vi "PCO_GetDeviceStatus.vi"(8 "error in (no error)":errorcluster {"code" format="%x"}, 10 "wNum":u16, 11 "ph":u64) -> (0 "error out":errorcluster {"code" format="%x"}, 1 "dwStatus":u32[](array[numeric]) format="%x", 2 "ErrorMessage":i32 format="%x", 3 "ph out":u64)   [LabVIEW 2019, in "SDK.lvlib" / "CameraAccess.lvlib"]
doc: "Gets the device availability status. Also returns the generation count if an IEEE 1394 interface is connected.\n\n dwStatus[0]-> 0x80000000: Device is available (0: not available)\ndwStatus[1]-> Generation count for IEEE1394 (undefined for other interfaces)"
uses:
  CameraAccess.lvlib
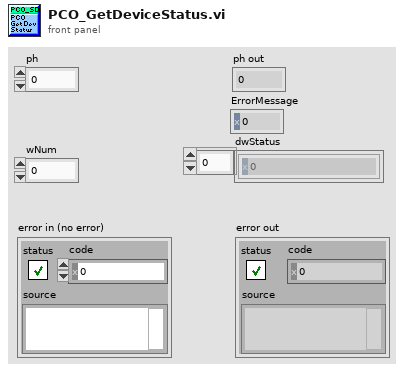
[diagram p1: front panel]
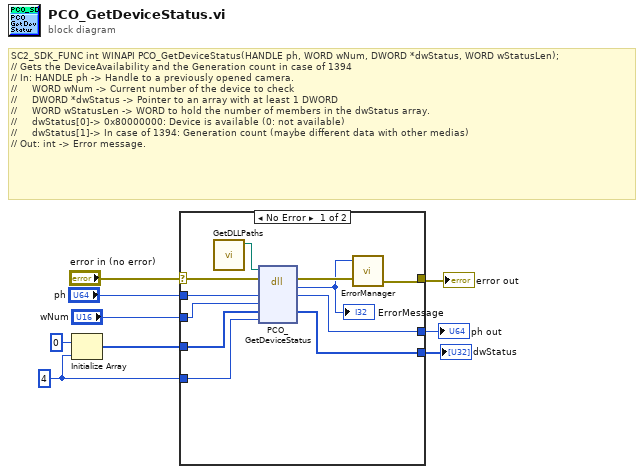
[diagram p0: block diagram]
diagram:
  w3 = u16 4 ("dimension size")
  # "SC2_SDK_FUNC int WINAPI PCO_GetDeviceStatus(HANDLE ph, WORD wNum, DWORD *dwStatus, WORD wStatusLen);\n// Gets the DeviceAvailability and the Generation count in case of 1394\n// In: HANDLE ph -> Handle to a previously opened camera.\n//     WORD wNum -> Current number of the device to check\n//     DWORD *dwStatus -> Pointer to an array with at least 1 DWORD\n//     WORD wStatusLen -> WORD to hold the number of members in the dwStatus array.\n//     dwStatus[0]-> 0x80000000: Device is available (0: not available)\n//     dwStatus[1]-> In case of 1394: Generation count (maybe different data with other medias)\n// Out: int -> Error message."
  n1 = Initialize Array(u32 0 ("element"), w3) -> (w4:u32[])
  n2 = case shown="No Error" "error in (no error)" {
    selector: "error in (no error)" -> [w19 w23]
    tunnel: [w20 w23] -> w9
    tunnel: [w16 w22] -> w7
    tunnel: "ph" -> [w15 w22]
    tunnel: w4 -> [w13 w21]
    tunnel: w3 -> [w12 _]
    tunnel: [w11 w21] -> w2
    tunnel: "wNum" -> [w10 _]
    frame No Error {
      n3 = call "GetDLLPaths.vi"() -> ("SC2_Cam_Path"=w14:path)  [unwired: 8 in, 3 out]
      n4 = dll-call lib="?" fn="PCO_GetDeviceStatus"(path in=w14, error in=w19, "ph"=w15, "wNum"=w10, "dwStatus"=w13, "wStatusLen"=w12) -> (error out=w18:errorcluster, "return type"=w17:i32, "ph"=w16:u64, "dwStatus"=w11:u32[])  [unwired: 3 in, 1 out]
      "ErrorMessage" <- w17
      n5 = call "ErrorManager.vi"("error in (no error)"=w18, "error code"=w17) -> ("error out"=w20:errorcluster)  [unwired: 2 in, 1 out]
    }
    frame Error {
    }
  }
  "error out" <- w9
  "ph out" <- w7
  "dwStatus" <- w2
